vi "testStringNotIncluded.vi"(9 "haystack":string, 10 "needle":string) -> (0 "error out":errorcluster)   [LabVIEW 2019, in "AssertionTest.lvlib" / "AssertStringNotContainsStringIgnoringCase.lvlib"]
uses:
  AssertStringNotContainsStringIgnoringCase.lvlib
  Assertion/Assertion.lvlib
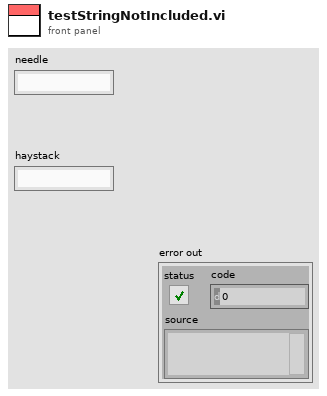
[diagram p1: front panel]
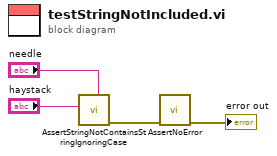
[diagram p0: block diagram]
diagram:
  n1 = call "AssertStringNotContainsStringIgnoringCase.vi"("Needle"="needle", "Haystack"="haystack") -> ("error out"=w1:errorcluster)  [unwired: 9 in]
  n2 = call "AssertNoError.vi"("error in (no error)"=w1) -> ("error out"=→"error out":errorcluster)  [unwired: 10 in]
